vi "Multitester.vi"() -> ()   [LabVIEW 2013]
uses:
  FA_LSSpecialTypes.ctl
  FA_LocalStore.lvlib
panel:
  in  "ID Array":string[](array[string])=["Id What?", "who", "why", "when", "where", "how"]
  out "XML String Array":string[](array[string])
  out "ETagArray":string[](array[string])
  in  "Error In":errorcluster
  in  "Special Type Array":T1[](array[typedef])
  out "Error Out":errorcluster
  in  "Delete Special Type":T1
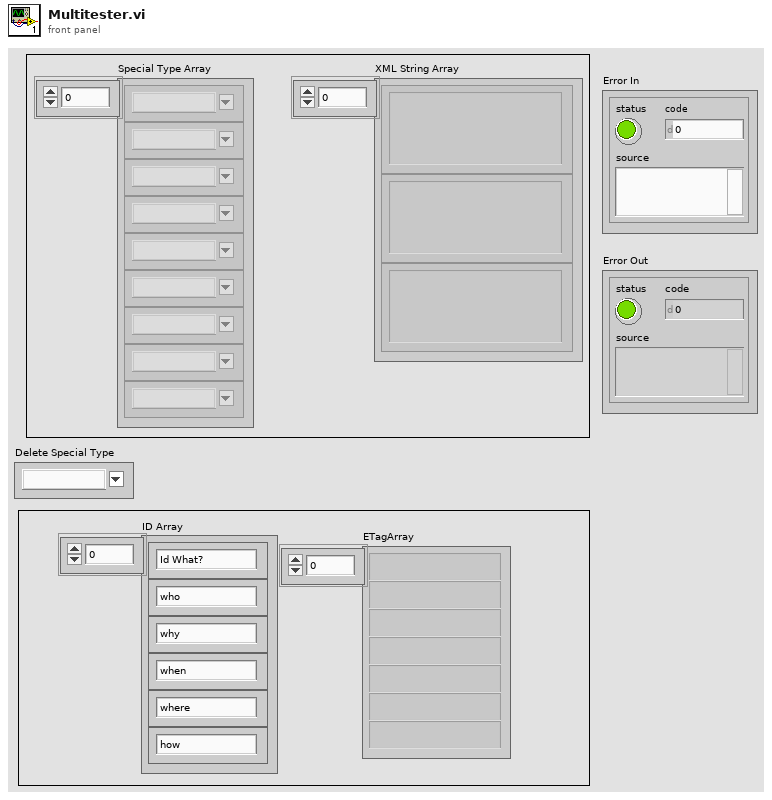
[diagram p1: front panel]
types:
  T1 = typedef "FA_LocalStore.lvlib/FA_LSSpecialTypes.ctl" = string
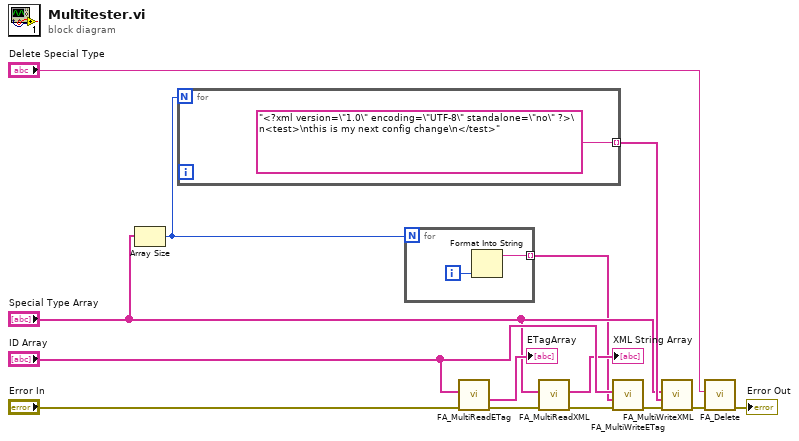
[diagram p0: block diagram]
diagram:
  n1 = Array Size(array="Special Type Array") -> (size(s)=w2:i32)
  n2 = for {
    N: w2 -> [_]
    tunnel: ["<?xml version=\"1.0\" encoding=\"UTF-8\" standalone=\"no\" ?>\n<test>\nthis is my next config change\n</test>" ("XML String")] -> w4 mode=indexing
  }
  n3 = for {
    N: w2 -> [_]
    tunnel: [w16] -> w1 mode=indexing
    i -> [w17]
    n4 = Format Into String(w17) -> (resulting string=w16:string)  [unwired: 3 in, 1 out]
  }
  n5 = call "FA_MultiReadETag.vi"("Error In"="Error In", "ID Array"="ID Array") -> ("Error Out"=w14:errorcluster, "ETagArray"=→"ETagArray":string[])  [unwired: 6 in]
  n6 = call "FA_MultiReadXML.vi"("Error In"=w14, "Special Type Array"="Special Type Array") -> ("Error Out"=w13:errorcluster, "XML String Array"=→"XML String Array":string[])  [unwired: 6 in]
  n7 = call "FA_MultiWriteETag.vi"("Error In"=w13, "eTag Array"=w1, "ID Array"="ID Array") -> ("Error Out"=w12:errorcluster)  [unwired: 6 in]
  n8 = call "FA_MultiWriteXML.vi"("Error In"=w12, "XML String Array"=w4, "Special Type Array"="Special Type Array") -> ("Error Out"=w11:errorcluster)  [unwired: 6 in]
  n9 = call "FA_Delete.vi"("Error In"=w11, "Special Type"="Delete Special Type") -> ("Error Out"=→"Error Out":errorcluster)  [unwired: 7 in]
